vi "Degrees to Radians.vi"   [LabVIEW 2017, in "NI_AngleManipulation.lvlib"]
doc: "Converts an angle from degrees to radians."
uses:
  <vilib>/Utility/AngleManip/NI_AngleManipulation.lvlib
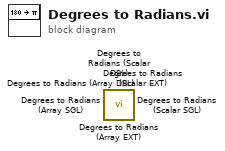
[diagram p0: block diagram]
diagram:
  n1 = call <vilib>:"Degrees to Radians (Array EXT).vi"() -> ()  [unwired: 3 in, 1 out]
  n2 = call <vilib>:"Degrees to Radians (Scalar EXT).vi"() -> ()  [unwired: 3 in, 1 out]
  n3 = call <vilib>:"Degrees to Radians (Array SGL).vi"() -> ()  [unwired: 3 in, 1 out]
  n4 = call <vilib>:"Degrees to Radians (Scalar SGL).vi"() -> ()  [unwired: 3 in, 1 out]
  n5 = call <vilib>:"Degrees to Radians (Array DBL).vi"() -> ()  [unwired: 3 in, 1 out]
  n6 = call <vilib>:"Degrees to Radians (Scalar DBL).vi"() -> ()  [unwired: 3 in, 1 out]
